vi "PowerGuardSetOverVoltage.vi"(0 "error in (no error)":errorcluster, 2 "Over Voltage":dbl=-1.0, 3 "Device In":u64) -> (7 "error out":errorcluster, 10 "Device Out":u64)   [LabVIEW 2020, in "Phidget Power Guard.lvlib"]
doc: "${OverVoltage:Header}"
uses:
  <instrlib>/Phidgets/Phidget Power Guard/Phidget Power Guard.lvlib
  <instrlib>/Phidgets/Phidget Common/Phidget Common.lvlib
  phidget22.dll
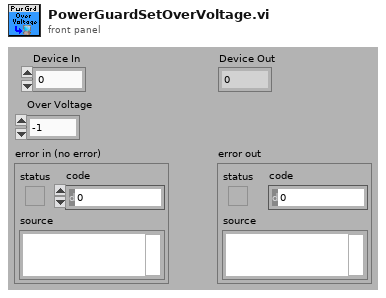
[diagram p1: front panel]
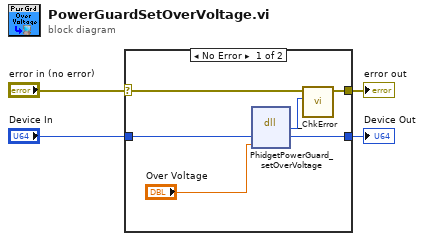
[diagram p0: block diagram]
diagram:
  n1 = case shown="No Error" "error in (no error)" {
    selector: "error in (no error)" -> [w8 w12]
    tunnel: [w7 w12] -> w3
    tunnel: "Device In" -> [w10 w11]
    tunnel: [w9 w11] -> w1
    frame No Error {
      n2 = dll-call lib="phidget22.*" fn="PhidgetPowerGuard_setOverVoltage"("phid"=w10, "overVoltage"="Over Voltage") -> ("return type"=w6:i32, "phid"=w9:u64)  [unwired: 4 in, 2 out]
      n3 = call <instrlib>:"_ChkError.vi"("Return Code"=w6, "error in (no error)"=w8) -> ("error out"=w7:errorcluster)  [unwired: 9 in]
    }
    frame Error {
    }
  }
  "error out" <- w3
  "Device Out" <- w1
